vi "CSV Name Change.vi"() -> ()   [LabVIEW 2022 SP3]
panel:
  out "Array":string[](array[string])
  in  "Folder Path":path
  out "All Folders":path[](array[path])
  out "All Files in Dir":path[](array[path])
  out "dup Folder Path":path
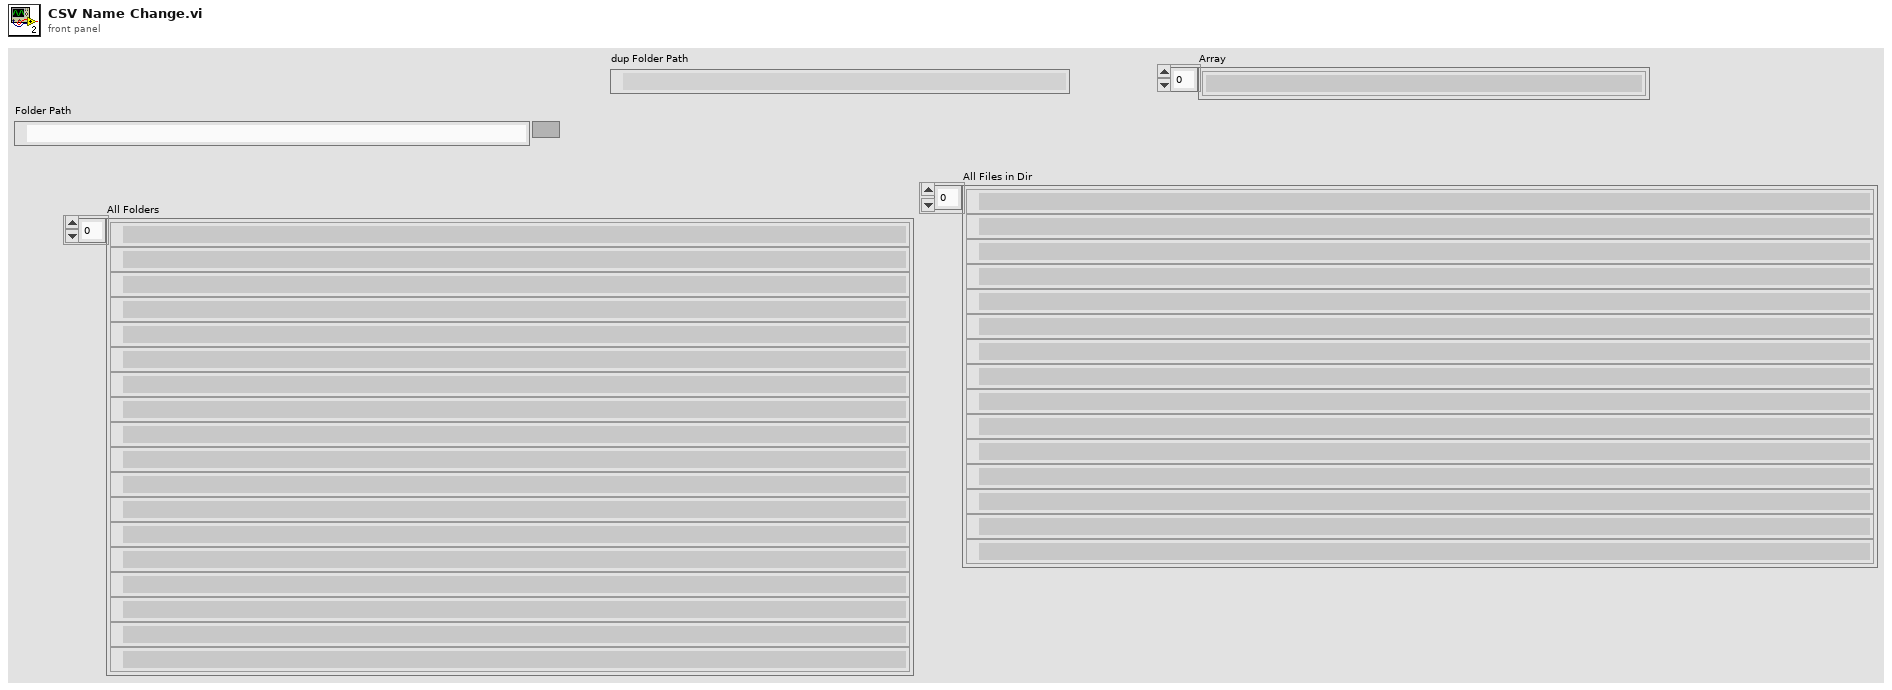
[diagram p1: front panel]
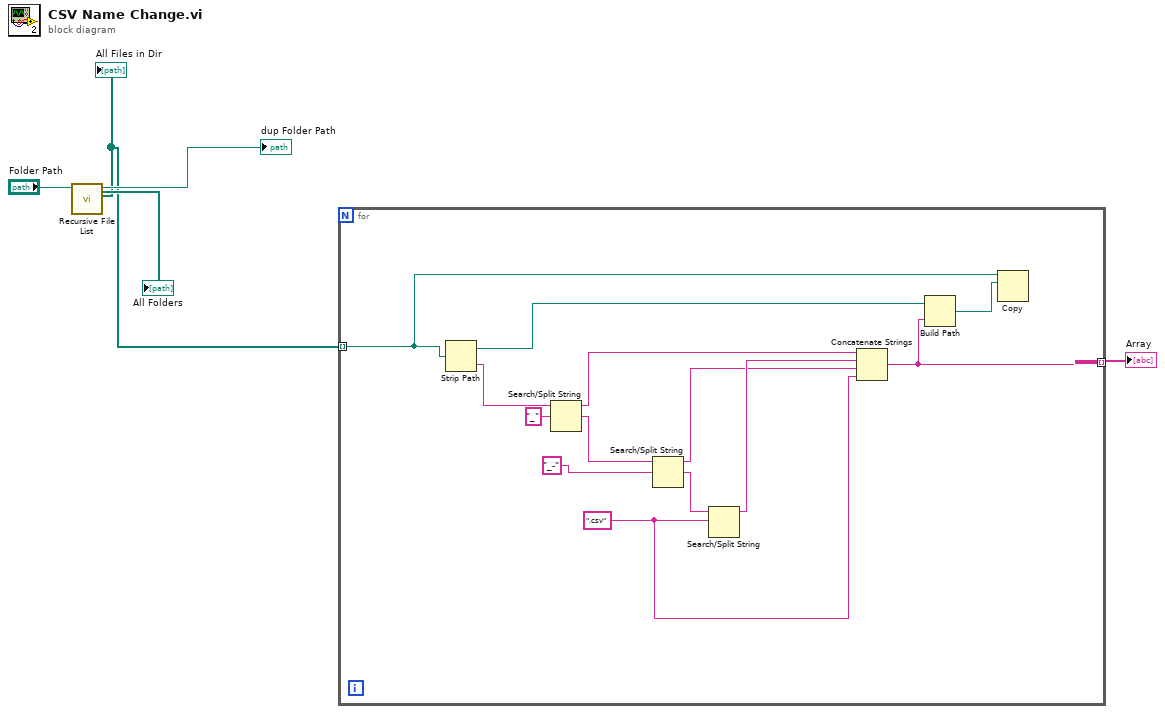
[diagram p0: block diagram]
diagram:
  n1 = call <vilib>:"Recursive File List.vi"("Folder Path"="Folder Path") -> ("All Files in Dir"=w2:path[], "dup Folder Path"=→"dup Folder Path":path, "All Folders"=→"All Folders":path[])  [unwired: 6 in, 2 out]
  "All Files in Dir" <- w2
  n2 = for {
    tunnel: w2 -> [w6] mode=indexing
    tunnel: [w9] -> w1 mode=indexing
    w10 = ".csv" ("search string/char (-)")
    n3 = Strip Path(path=w6) -> (stripped path=w8:path, name=w18:string)
    n4 = Search/Split String(string=w18, search string/char (-)="_") -> (substring before match=w14:string, match + rest of string=w16:string)  [unwired: 1 in, 1 out]
    n5 = Search/Split String(string=w16, search string/char (-)="_-") -> (substring before match=w11:string, match + rest of string=w13:string)  [unwired: 1 in, 1 out]
    n6 = Search/Split String(string=w13, search string/char (-)=w10) -> (substring before match=w12:string)  [unwired: 1 in, 2 out]
    n7 = Concatenate Strings(w14, w12, w11, w10) -> (w9:string)
    n8 = Build Path(base path=w8, name or relative path=w9) -> (appended path=w7:path)
    n9 = Copy(10:w7, 11:w6) -> ()  [unwired: 3 in, 3 out]
  }
  "Array" <- w1
